vi "throttle.vi"(11 "x":dbl) -> (3 "x/y":dbl)   [LabVIEW 2013]
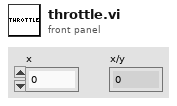
[diagram p1: front panel]
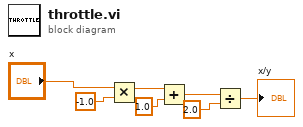
[diagram p0: block diagram]
diagram:
  n1 = Multiply(x="x", y=-1.0) -> (x*y=w2:dbl)
  n2 = Add(x=w2, y=1.0) -> (x+y=w4:dbl)
  n3 = Divide(x=w4, y=2.0) -> (x/y=→"x/y":dbl)
